vi "While Loop Synchronization.vi"() -> ()   [LabVIEW 2023]
doc: "Demonstrates the use of the Synchronize to Scan Engine VI to synchronize a While Loop to the period of the NI Scan Engine. This VI also checks for lateness and allows you to choose whether to set a major or minor fault upon detecting a late loop iteration."
panel:
  in  "Stop":bool
  out "Loop Iterations":i32
  out "Loop Late?":bool
  in  "Make Fault Major?":bool
  in  "Generate Fault on Late Loop Iterations?":bool
  in  "Wait Amount (ms)":u32(slide)=25 scale=0.0..250.0
  in  "Scan Period (ms)":u32=100
  # "Overview: Sets the period of the NI Scan Engine and uses the Synchronize to Scan Engine VI to synchronize a While Loop to the period of the NI Scan Engine.  This VI also checks for lateness and allows you to choose whether to set a major or minor fault upon detecting a late loop iteration.  \nRequirements: LabVIEW Real-Time Module and NI-RIO driver\nInstructions:\n1. In Measurement & Automation Explorer, ensure that LabVIEW Real-Time and the NI Scan Engine are installed on your RT target.\n2. From the Project Explorer window, set the IP address of your RT target.\n3. Set the Scan Period (ms) front panel control of either the Timed Loop Synchronization.vi or While Loop Synchronization.vi to the desired loop rate. \n4. Run the VI in which you chose to set the Scan Period (mSec) control. \n5. Use the controls on the front panel to increase the wait amount in the While Loop. When you increase the wait amount beyond the scan period, the loop runs late and LabVIEW generates a fault.\n6. Run Fault Monitor.vi.\n7. Use the controls on the front panel to clear a specific fault code or to clear all faults.\n8. Click the Stop buttons on both VIs."
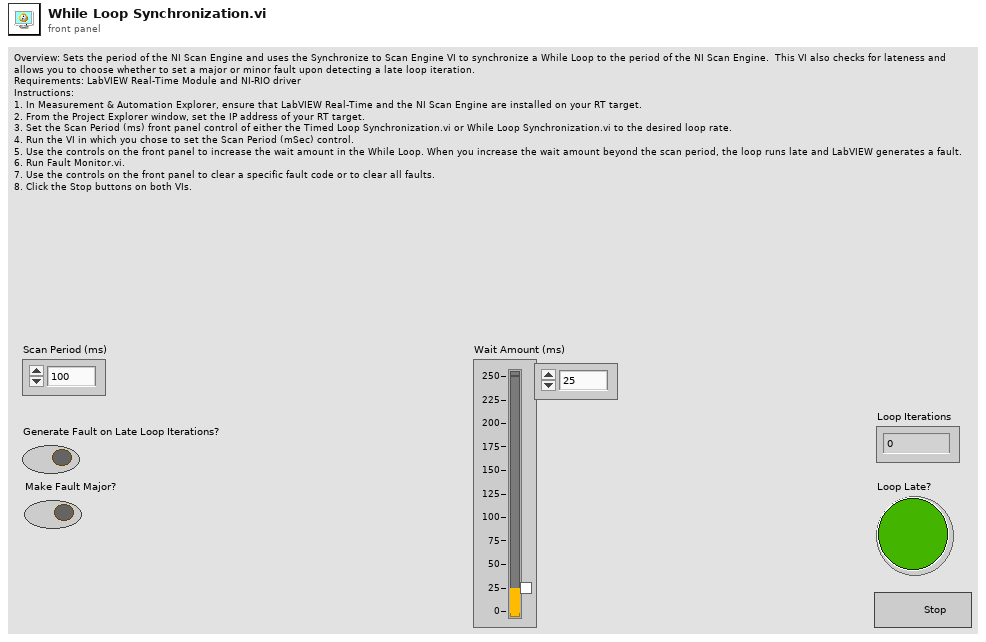
[diagram p1: front panel]
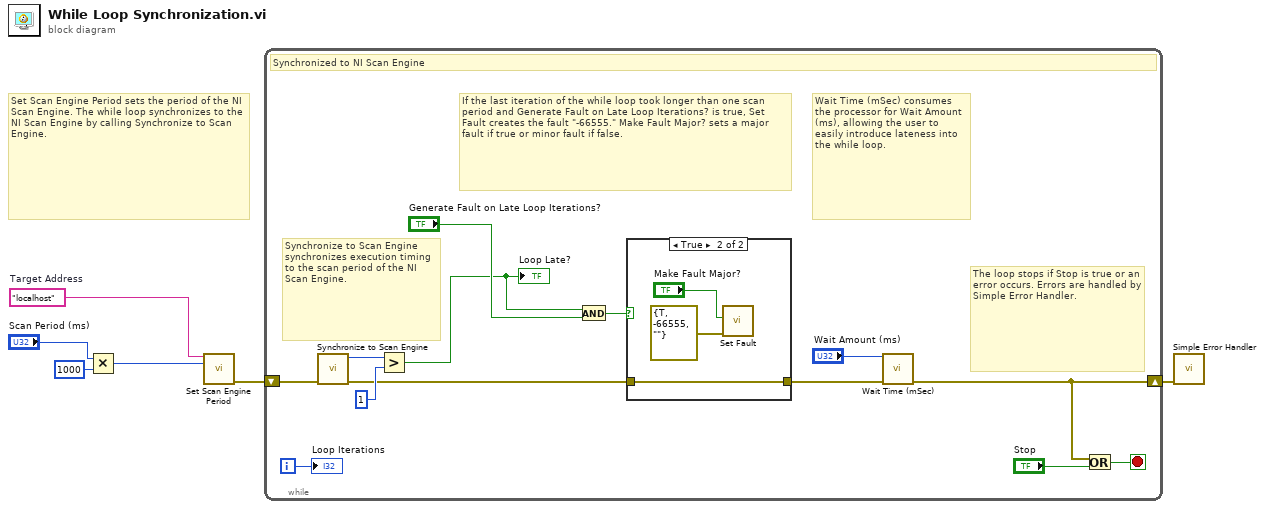
[diagram p0: block diagram]
diagram:
  w4 = "localhost"  # Target Address
  # "Set Scan Engine Period sets the period of the NI Scan Engine. The while loop synchronizes to the NI Scan Engine by calling Synchronize to Scan Engine."
  n1 = Multiply(x="Scan Period (ms)", y=u32 1000) -> (x*y=w5:u32)
  n2 = call <vilib>:"Set Scan Engine Period.vi"("target address (localhost)"=w4, "scan period (uSec)"=w5) -> ("error out"=w2:errorcluster)  [unwired: 1 in, 12 out]
  n3 = while {
    shift-right: [w14] -> w1
    shift-left: w2 -> [w9]
    i -> [w19]
    stop <- w12 stop-if-true
    # "Synchronize to Scan Engine synchronizes execution timing to the scan period of the NI Scan Engine."
    # "The loop stops if Stop is true or an error occurs. Errors are handled by Simple Error Handler."
    # "Wait Time (mSec) consumes the processor for Wait Amount (ms), allowing the user to easily introduce lateness into the while loop."
    # "If the last iteration of the while loop took longer than one scan period and Generate Fault on Late Loop Iterations? is true, Set Fault creates the fault \"-66555.\" Make Fault Major? sets a major fault if true or minor fault if false."
    # "Synchronized to NI Scan Engine"
    n4 = call <vilib>:"Synchronize to Scan Engine.vi"("error in (no error)"=w9) -> ("error out"=w8:errorcluster, "scans since last call"=w10:u32)  [unwired: 9 out]
    n5 = Greater?(x=w10, y=u32 1) -> (0:w7:bool)
    "Loop Late?" <- w7
    n6 = And(x=w7, y="Generate Fault on Late Loop Iterations?") -> (x .and. y?=w18:bool)
    n7 = case shown="True" w18 {
      tunnel: w8 -> [w20 w21]
      tunnel: [w20 w21] -> w15
      frame False {
      }
      frame True {
        n8 = call <vilib>:"Set Fault.vi"("error in (user fault)"=errorcluster {"status"=TRUE, "code"=-66555, "source"=""}, "major fault (F)"="Make Fault Major?") -> ()  [unwired: 10 out]
      }
    }
    n9 = call "Wait Time (mSec).vi"("error in"=w15, "Spin Amount (mS)"="Wait Amount (ms)") -> ("error out"=w14:errorcluster)  [unwired: 9 in]
    n10 = Or(x=w14, y="Stop") -> (x .or. y?=w12:bool)
    "Loop Iterations" <- w19
  }
  n11 = call <vilib>:"Simple Error Handler.vi"("error in (no error)"=w1) -> ()  [unwired: 1 in, 8 out]
